vi "Control Panel No Objects.vi"(8 "error in (no error)":errorcluster) -> (0 "error out":errorcluster)   [LabVIEW 2009]
doc: "(Dynamic) A user-level application that simulates the physical front panel of the Instrument. Provide the user with buttons to manually control features of the instrument, and provide indicators of its current state."
uses:
  Areas.ctl
  Utility Classes/Readable/Channel Names.ctl
  Utility Classes/Readable/Channel Units.ctl
  Global/GPIB Numbers.vi
  <vilib>/Utility/error.llb/DialogType.ctl
  Spectrometer/JY-SPEX-TRIAX/controls.llb/Slits.ctl
  Synapse CCD.lvclass
  File IO/File IO.lvclass
  Spectrometer/JY-SPEX-TRIAX/JY-SPEX-TRIAX.lvlib
  Utility Classes/Readable/Readable.lvclass
panel:
  out "Resolution\n(nm/pixel)":dbl[unit] format="%#_3g"
  in  "File Name":path
  in  "Comments":string
  in  "Export\nPlot":bool
  in  "Cosmic Ray\nRemoval?":bool
  out "UnProcessed Spectra":T1(graph)
  in  "# to Average":u32
  in  "Averaging?":bool
  in  "Time Between Acq. (ms)":u32
  out "Spectrum":cluster{"Ramp Pattern":dbl[], "X array":dbl[]}[](graph)
  out "CCD State":string
  in  "Take Spectra":bool
  in  "Set CCD":bool
  in  "Set Grating":bool
  in  "stop":bool
  in  "Exit Slit":dbl[unit]
  in  "Entrance Slit":dbl[unit]
  out "Min":dbl[unit]
  out "Max":dbl[unit]
  in  "Center Wavelength":dbl[unit]
  in  "Grating":u16(ring) items=["1200 lines/mm - 500 nm Blaze", "1200 lines/mm - 750 nm Blaze", "600 lines/mm - 1000 nm Blaze"]
  in  "GAIN":u16(ring) caption="Device Name" items=["High Light", "Best Dynamic", "High Sensitivity"]
  in  "ADC":u16(ring) caption="Device Name" items=["   20 kHz", "1 MHz", "1 MHz Ultra"]
  in  "Integration time":dbl[unit]=0.01
  in  "Dark Subtract?":bool
  in  "Copy Actual to Set":bool
  in  "Populate Fields with Member Data":bool
  # "Must Set CCD after any change in this box"
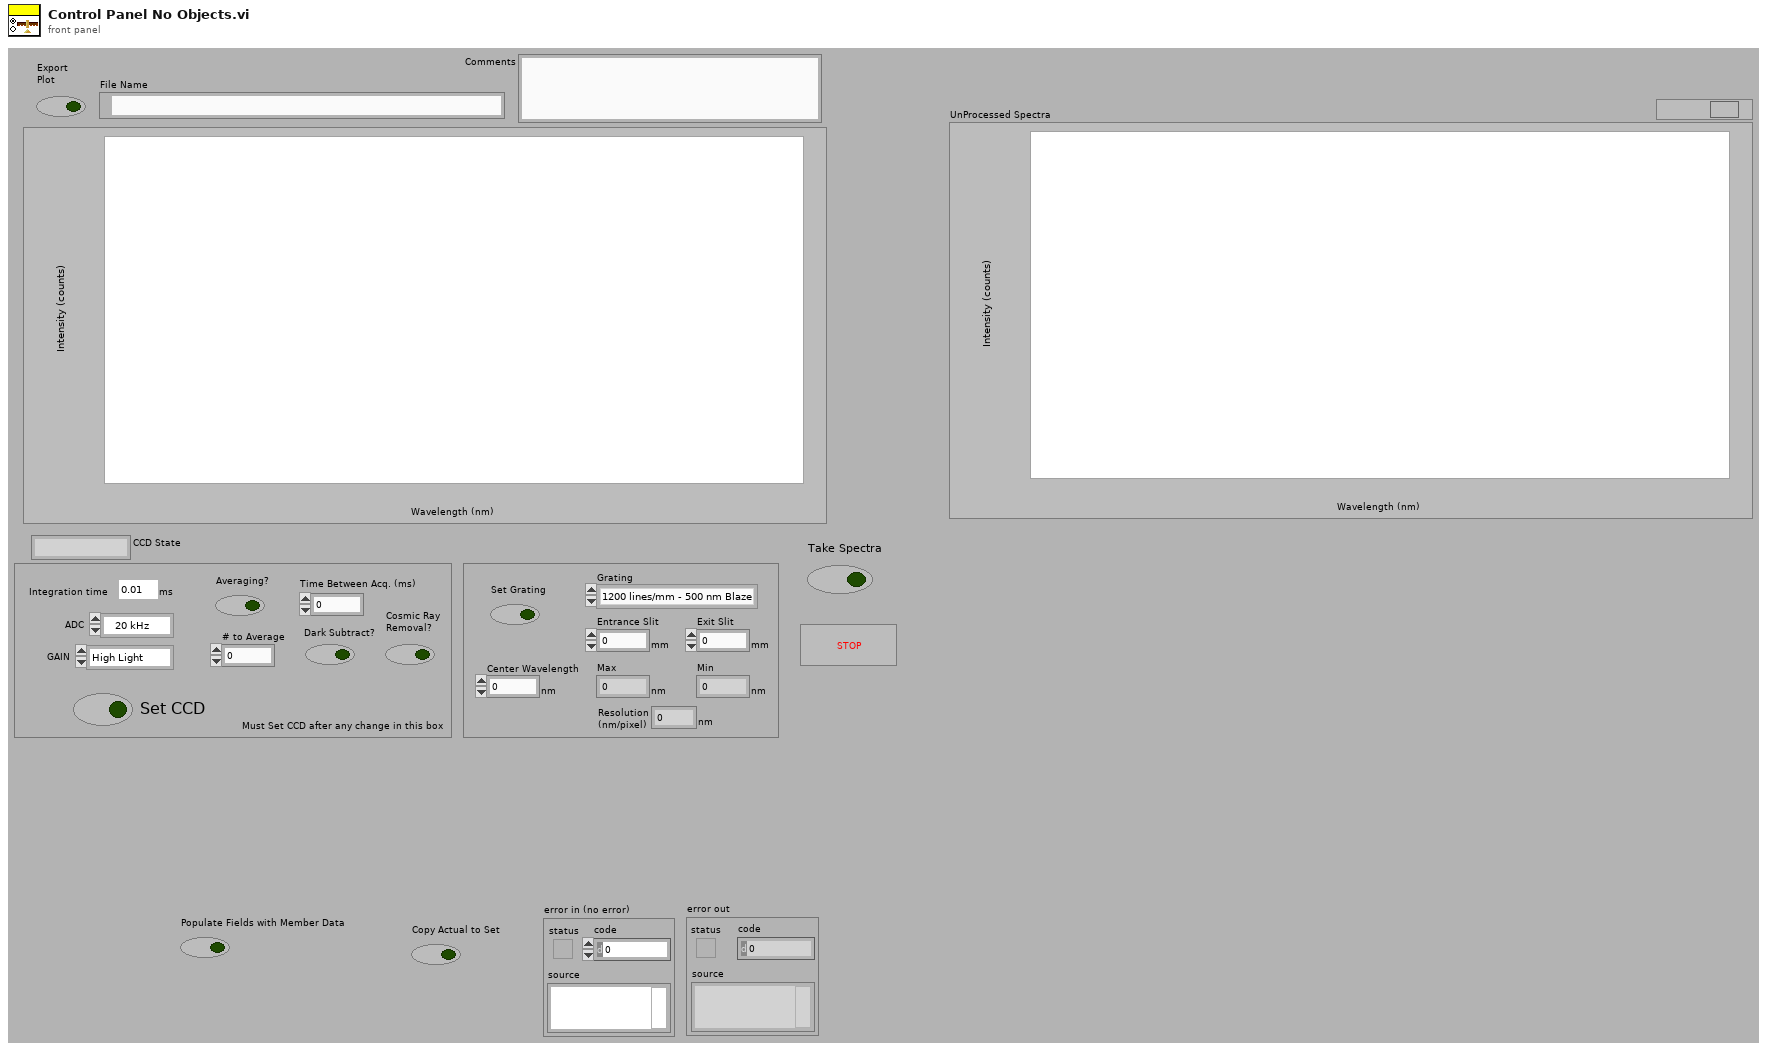
[diagram p1: front panel]
types:
  T1 = cluster{"Array of Wavelengths":dbl[], "Raw Data":i32[]}[]
  T2 = typedef "Synapse CCD.lvclass/Areas.ctl" = i32[][]
  T3 = typedef "Readable.lvclass/Channel Names.ctl" = string[]
  T4 = typedef "Readable.lvclass/Channel Units.ctl" = string[]
  T5 = cluster{"JYCCDLib.IJYCCDReqd":refnum<k7>, "JYMONOLib.IJYMonoReqd":refnum<k7>, "Integration time":dbl[unit], "ADC":u16, "GAIN":u16, "Areas":T2, "Most Recent Data Object":refnum<k7>, "Mono Properties":cluster{"Grating":u16, "Center Wavelength":dbl[unit], "Entrance Slit":dbl[unit], "Exit Slit":dbl[unit]}, "Coverage":cluster{"Max":dbl[unit], "Min":dbl[unit]}, "Multi-Acquisitions":cluster{"Dark Subtract?":bool, "Averaging?":bool, "Cosmic Ray Removal?":bool, "# to Average":u32, "Time Between Acq.":u32, "Acquisitions Control Array":bool[], "Raw Data":i32[][], "Processed Data":dbl[], "Array of Wavelengths":dbl[]}, "Channel Names":T3, "Channel Units":T4}
  T6 = typedef "DialogType.ctl" = u16
  T7 = typedef "GPIB Type Def.ctl" = cluster{"Name":string, "bus":dbl, "GPIB":dbl, "GPIB as string":string, "byte":i32, "VISA Resource Name":refnum<visa-resource-name>}
  T8 = typedef "JY-SPEX-TRIAX.lvlib/Slits.ctl" = enum16{"0 (Front/Axial Entrance)", "1 (Side/Lateral Entrance)", "2 (Front/Axial Exit)", "3 (Side/Lateral Exit)"}
  T9 = cluster{"Array of Wavelengths":dbl[], "Raw Data":i32[]}
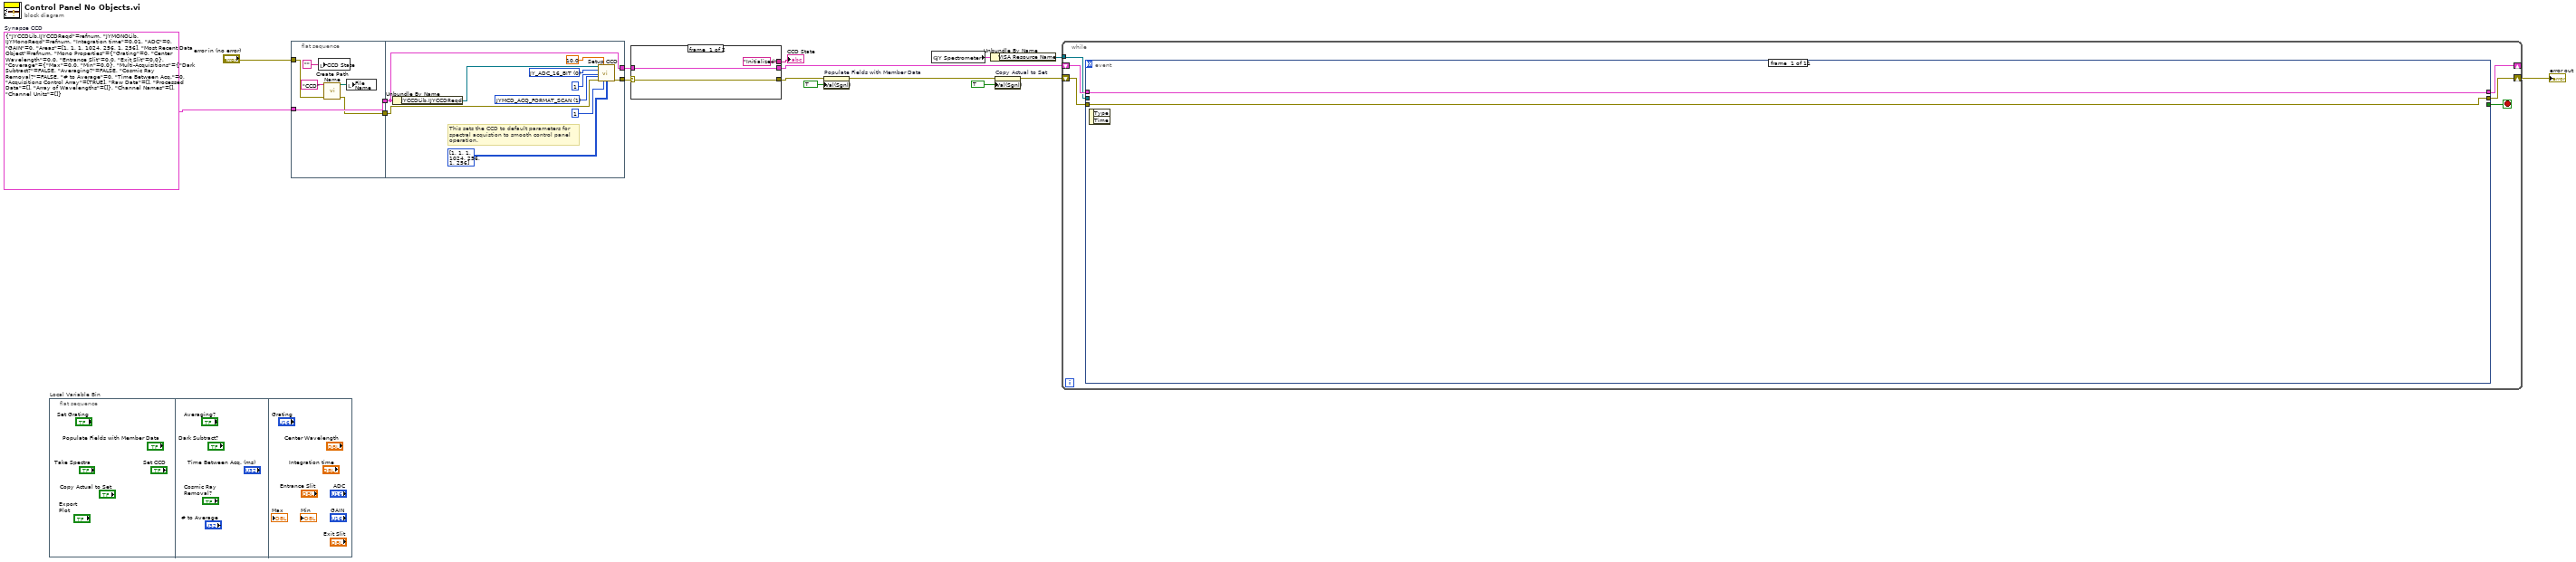
[diagram p0: block diagram]
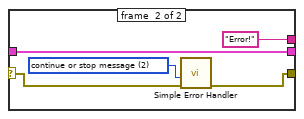
[diagram p2: hidden frame]
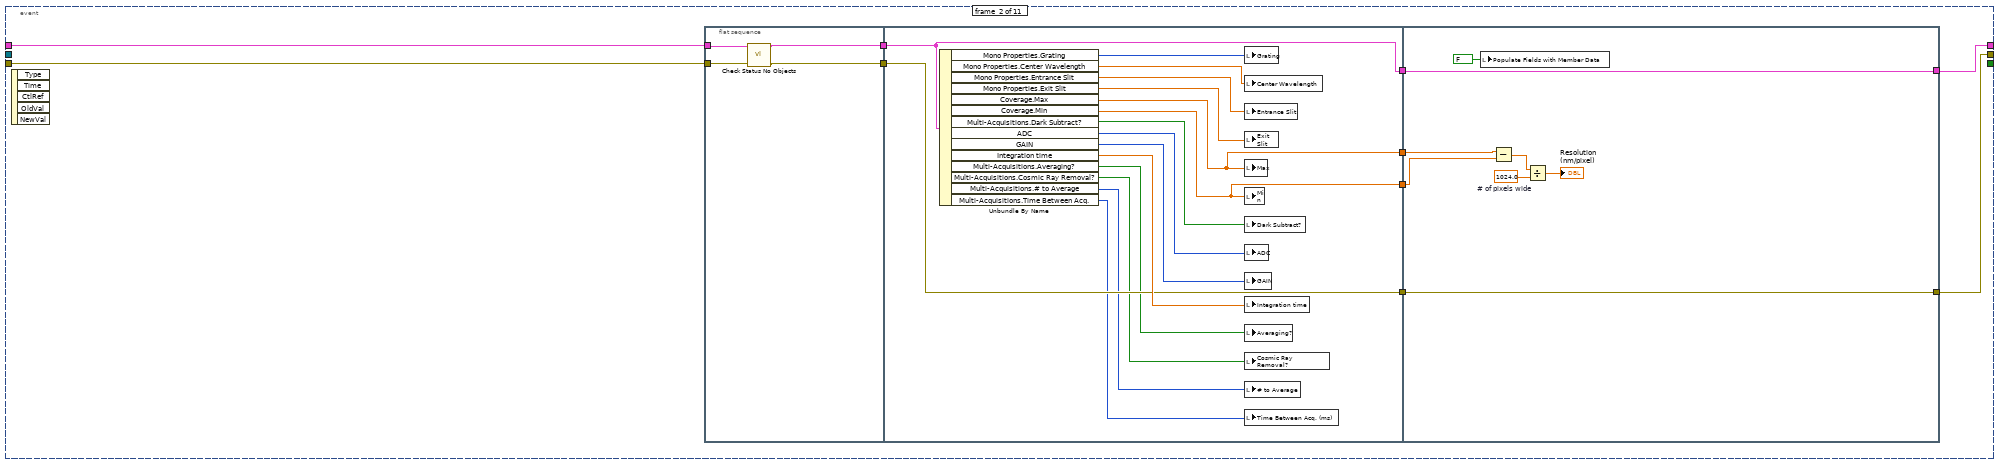
[diagram p3: hidden frame]
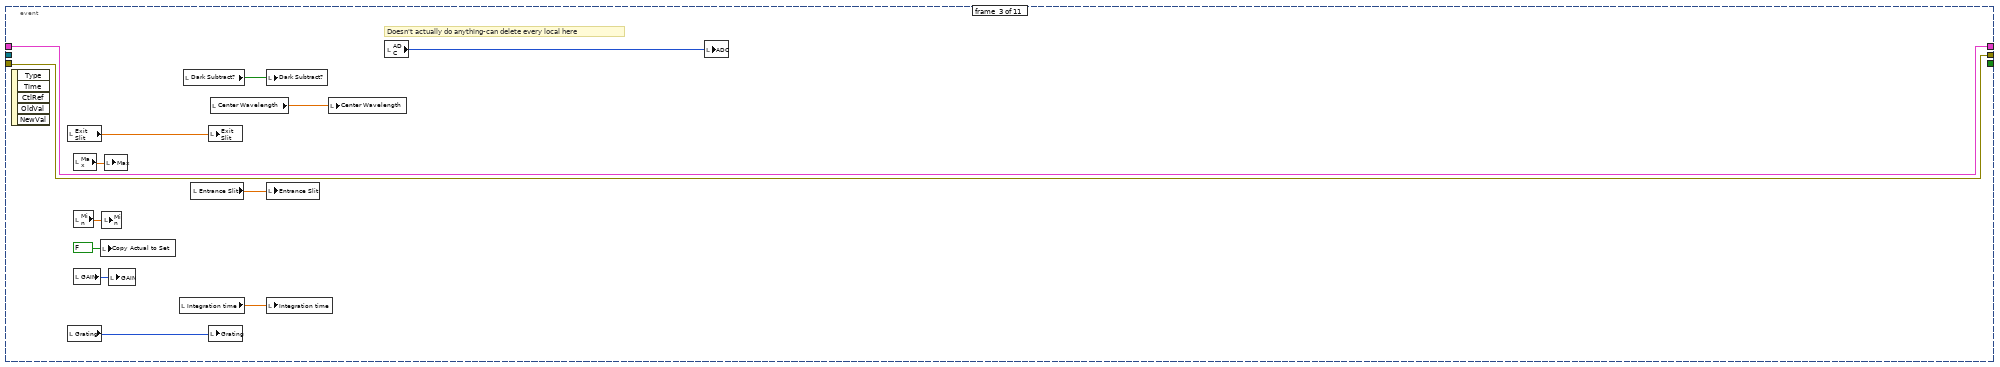
[diagram p4: hidden frame]
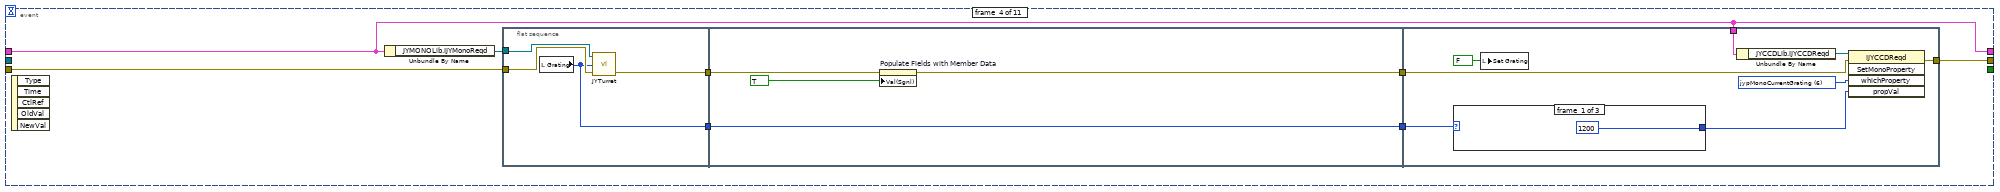
[diagram p5: hidden frame]
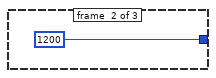
[diagram p6: hidden frame]
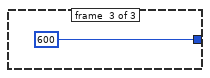
[diagram p7: hidden frame]
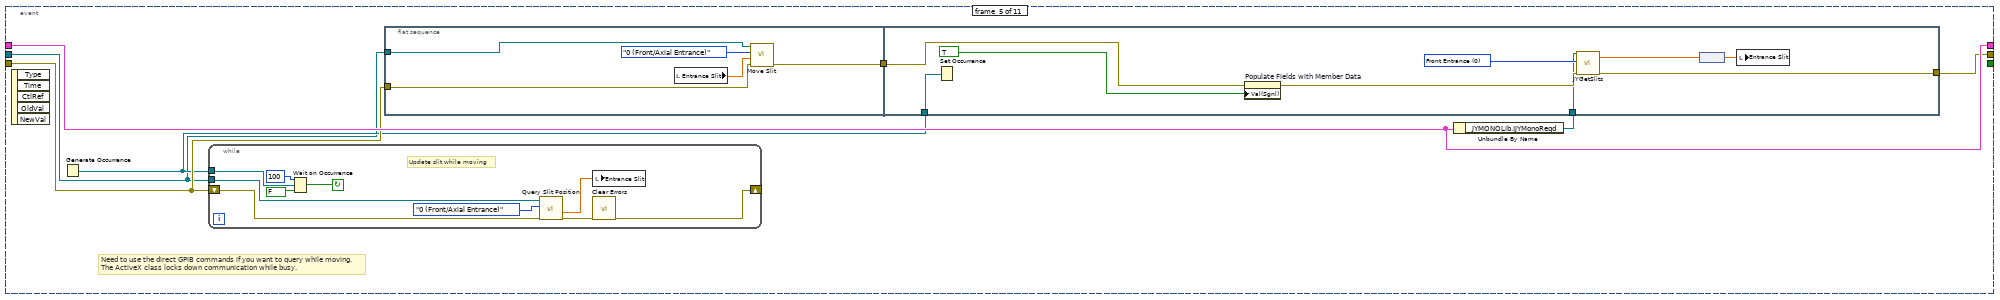
[diagram p8: hidden frame]
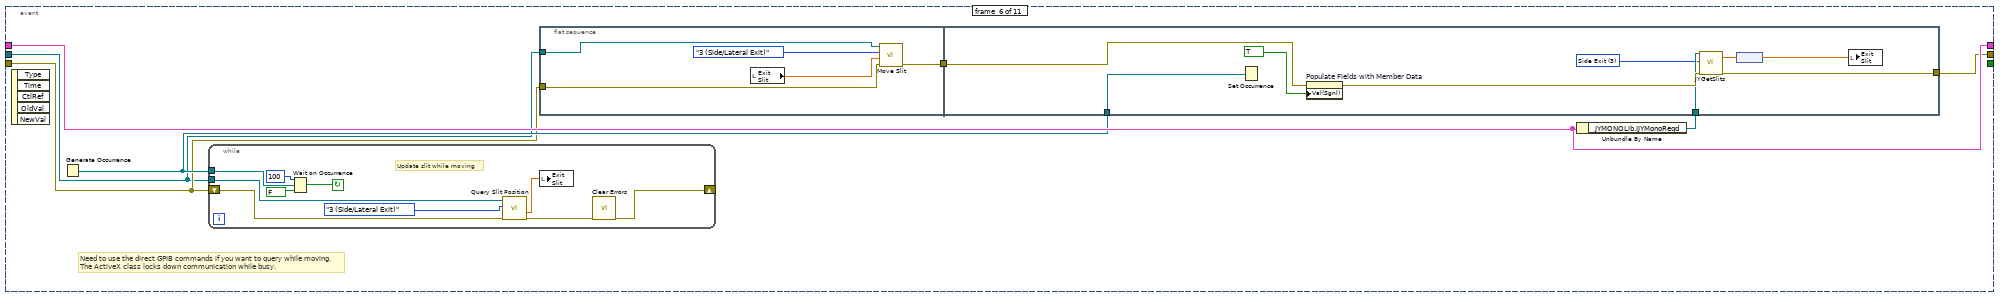
[diagram p9: hidden frame]
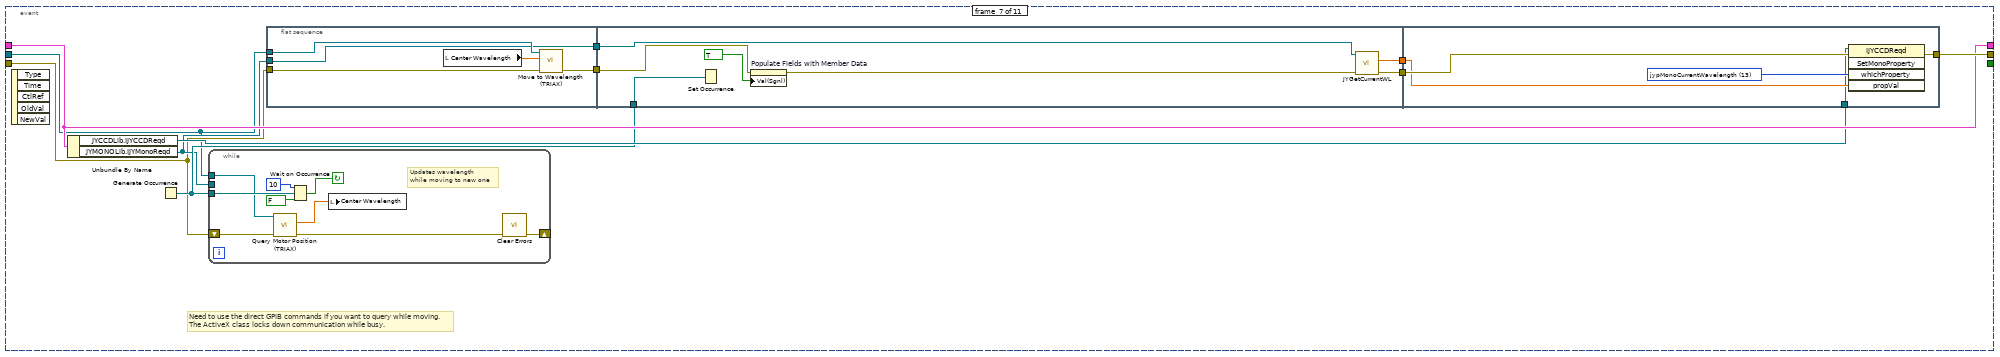
[diagram p10: hidden frame]
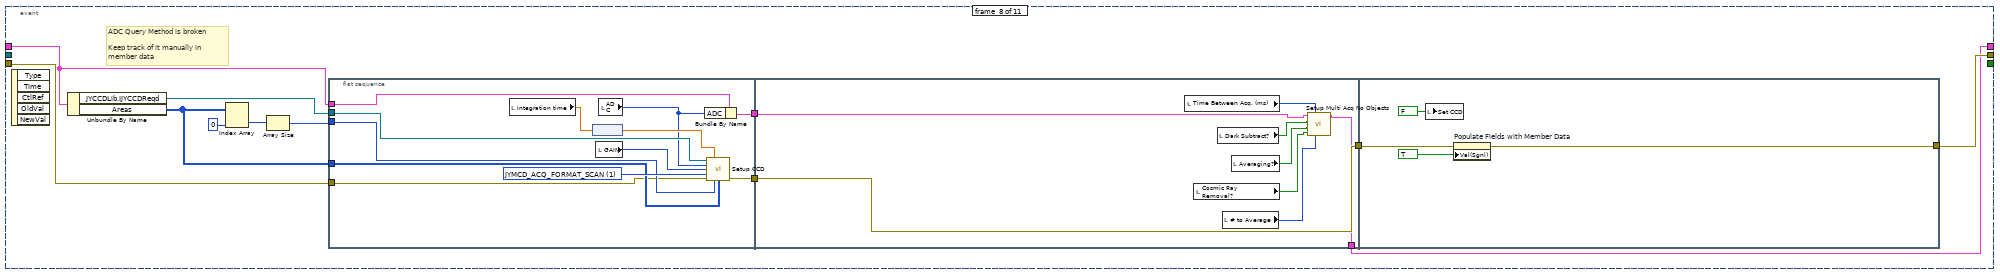
[diagram p11: hidden frame]
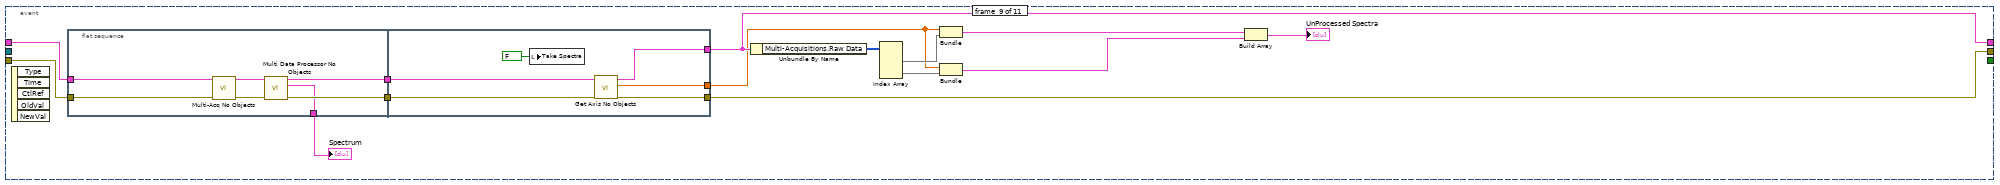
[diagram p12: hidden frame]
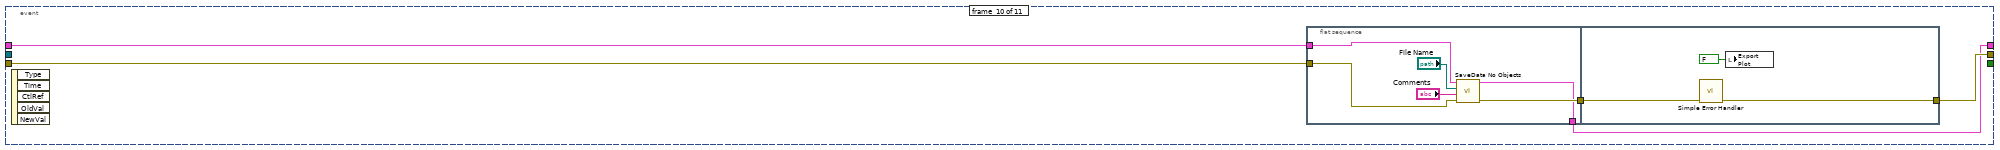
[diagram p13: hidden frame]
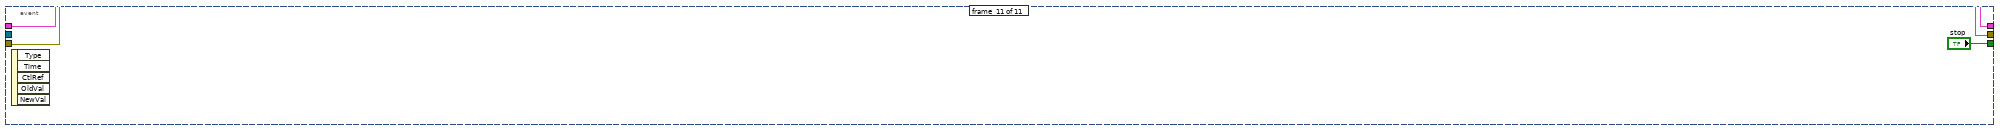
[diagram p14: hidden frame]
diagram:
  w3 = T5 {"JYCCDLib.IJYCCDReqd"=refnum, "JYMONOLib.IJYMonoReqd"=refnum, "Integration time"=0.01, "ADC"=0, "GAIN"=0, "Areas"=[[1, 1, 1, 1024, 256, 1, 256]], "Most Recent Data Object"=refnum, "Mono Properties"={"Grating"=0, "Center Wavelength"=0.0, "Entrance Slit"=0.0, "Exit Slit"=0.0}, "Coverage"={"Max"=0.0, "Min"=0.0}, "Multi-Acquisitions"={"Dark Subtract?"=FALSE, "Averaging?"=FALSE, "Cosmic Ray Removal?"=FALSE, "# to Average"=0, "Time Between Acq."=0, "Acquisitions Control Array"=[TRUE], "Raw Data"=[], "Processed Data"=[], "Array of Wavelengths"=[]}, "Channel Names"=[], "Channel Units"=[]}  # Synapse CCD
  n1 = flat-sequence "Local Variable Bin" {
    frame #0 {
    }
    frame #1 {
    }
    frame #2 {
    }
  }
  n2 = flat-sequence {
    tunnel: "error in (no error)" -> [w22]
    tunnel: [w18] -> w7
    tunnel: w3 -> [w18]
    tunnel: [w17] -> w2
    tunnel: [w32] -> w11
    tunnel: [w23] -> w12
    tunnel: w7 -> [w32]
    tunnel: w2 -> [w26]
    frame #0 {
      n3 = local write "CCD State"("") -> ()
      n4 = call "Create Path Name.vi"("error in"=w22, "filename"="CCD") -> ("error out"=w17:errorcluster, "path"=w20:path)  [unwired: 4 out]
      n5 = local write "File Name"(w20) -> ()
    }
    frame #1 {
      w27 = 1 items=["JYMCD_ACQ_FORMAT_IMAGE", "JYMCD_ACQ_FORMAT_SCAN"] ("Acquisition type")
      w29 = 0 items=["JY_ADC_16_BIT", "JY_ADC_14_BIT", "JY_ADC_18_BIT"] ("Select ADC")
      # "This sets the CCD to default parameters for\nspectral acquistion to smooth control panel\noperation."
      n6 = Unbundle By Name(w32) -> ("JYCCDLib.IJYCCDReqd"=w31:refnum<k7>)
      n7 = call "Setup CCD.vi"("IJYCCDReqd In"=w31, "Integration time(ms)"=10.0 ("IntegrationTime"), "Select ADC"=w29, "Gain"=1, "Acquisition type"=w27, "error in (no error)"=w26, "numAreas"=1, "areas :"=T2 [[1, 1, 1, 1024, 256, 1, 256]] ("Areas")) -> ("error out"=w23:errorcluster)  [unwired: 5 in, 2 out]
    }
  }
  n8 = case shown="No Error" w12 {
    selector: w12 -> [w34 w38]
    tunnel: w11 -> [w35 w40]
    tunnel: [w35 w40] -> w10
    tunnel: [w34 w37] -> w9
    tunnel: ["Initialized" ("String") "Error!" ("String")] -> w8
    frame #0 {
    }
    frame #1 {
      w36 = T6 2 items=["no dialog", "OK message", "continue or stop message", "OK message + warnings", "continue/stop + warnings"] ("type of dialog (OK msg:1)")
      n9 = call <vilib>:"Simple Error Handler.vi"("type of dialog (OK msg:1)"=w36, "error in (no error)"=w38) -> ("error out"=w37:errorcluster)  [unwired: 3 in, 4 out]
    }
  }
  "CCD State" <- w8
  n10 = property on="Populate Fields with Member Data" class="Bool (strict)"(error in=w9, "Val(Sgnl)"=TRUE ("Value (Signaling)")) -> (error out=w16:errorcluster)  [unwired: 1 in, 1 out]
  n11 = global read "GPIB Numbers.vi" "JY Spectrometer"() -> (w6:T7)
  n12 = Unbundle By Name(w6) -> ("VISA Resource Name"=w5:refnum<visa-resource-name>)
  n13 = property on="Copy Actual to Set" class="Bool (strict)"(error in=w16, "Val(Sgnl)"=TRUE ("Value (Signaling)")) -> (error out=w15:errorcluster)  [unwired: 1 in, 1 out]
  n14 = while {
    shift-right: [w44] -> w1
    shift-left: w15 -> [w45]
    shift-right: [w43] -> _
    shift-left: w10 -> [w46]
    tunnel: w5 -> [w41]
    stop <- w42 stop-if-true
    n15 = event shown="[9] \"Export\nPlot\": Value Change" {
      selector: _ -> [_ _ _ _ _ _ _ _ _ _ _]
      dyn-events: _ -> [_ _ _ _ _ _ _ _ _ _ _]
      timeout: _ -> [_ _ _ _ _ _ _ _ _ _ _]
      tunnel: w46 -> [w48 w58 w88 w100 w132 w163 w195 w227 w271 w292 w304]
      tunnel: w45 -> [w47 w56 w89 w106 w130 w160 w190 w233 w275 w293 w303]
      tunnel: [w47 w55 w89 w105 w131 w162 w199 w232 w272 w291 w303] -> w44
      tunnel: [w48 w57 w88 w100 w132 w163 w195 w228 w270 w290 w304] -> w43
      tunnel: [_ _ _ _ _ _ _ _ _ _ "stop"] -> w42
      tunnel: w41 -> [_ _ _ _ w128 w158 w189 _ _ _ _]
      event #0 {
        n16 = event-data() -> ()  [unwired: 1 in, 2 out]
      }
      event #1 {
        n17 = event-data() -> ()  [unwired: 1 in, 5 out]
        n18 = flat-sequence {
          tunnel: w56 -> [w59]
          tunnel: w58 -> [w62]
          tunnel: [w61] -> w52
          tunnel: [w60] -> w51
          tunnel: [w70] -> w54
          tunnel: [w69] -> w53
          tunnel: w52 -> [w70]
          tunnel: w51 -> [w69]
          tunnel: [w64] -> w50
          tunnel: [w63] -> w49
          tunnel: [w85] -> w55
          tunnel: [w86] -> w57
          tunnel: w54 -> [w86]
          tunnel: w53 -> [w85]
          tunnel: w50 -> [w83]
          tunnel: w49 -> [w82]
          frame #0 {
            n19 = call "Check Status No Objects.vi"("error in (no error)"=w59, "Synapse CCD in"=w62) -> ("error out"=w60:errorcluster, "Synapse CCD out"=w61:T5)  [unwired: 6 in, 2 out]
          }
          frame #1 {
            n20 = Unbundle By Name(w70) -> ("Mono Properties.Grating"=w78:u16, "Mono Properties.Center Wavelength"=w77:dbl[unit], "Mono Properties.Entrance Slit"=w76:dbl[unit], "Mono Properties.Exit Slit"=w75:dbl[unit], "Coverage.Max"=w64:dbl[unit], "Coverage.Min"=w63:dbl[unit], "Multi-Acquisitions.Dark Subtract?"=w74:bool, "ADC"=w73:u16, "GAIN"=w72:u16, "Integration time"=w71:dbl[unit], "Multi-Acquisitions.Averaging?"=w65:bool, "Multi-Acquisitions.Cosmic Ray Removal?"=w66:bool, "Multi-Acquisitions.# to Average"=w67:u32, "Multi-Acquisitions.Time Between Acq."=w68:u32)
            n21 = local write "Grating"(w78) -> ()
            n22 = local write "Center Wavelength"(w77) -> ()
            n23 = local write "Entrance Slit"(w76) -> ()
            n24 = local write "Exit Slit"(w75) -> ()
            n25 = local write "Max"(w64) -> ()
            n26 = local write "Min"(w63) -> ()
            n27 = local write "Dark Subtract?"(w74) -> ()
            n28 = local write "ADC"(w73) -> ()
            n29 = local write "GAIN"(w72) -> ()
            n30 = local write "Integration time"(w71) -> ()
            n31 = local write "Averaging?"(w65) -> ()
            n32 = local write "Cosmic Ray\nRemoval?"(w66) -> ()
            n33 = local write "# to Average"(w67) -> ()
            n34 = local write "Time Between Acq. (ms)"(w68) -> ()
          }
          frame #2 {
            w80 = 1024.0  # # of pixels wide
            n35 = local write "Populate Fields with Member Data"(FALSE ("Populate Fields with Member Data")) -> ()
            n36 = Subtract(x=w83, y=w82) -> (x-y=w81:dbl[unit])
            n37 = Divide(x=w81, y=w80) -> (x/y=→"Resolution\n(nm/pixel)":dbl[unit])
          }
        }
      }
      event #2 {
        # "Doesn't actually do anything-can delete every local here"
        n38 = event-data() -> ()  [unwired: 1 in, 5 out]
        n39 = local read "Exit Slit"() -> (w94:dbl[unit])
        n40 = local read "Grating"() -> (w92:u16)
        n41 = local read "Max"() -> (w90:dbl[unit])
        n42 = local read "Min"() -> (w96:dbl[unit])
        n43 = local read "GAIN"() -> (w93:u16)
        n44 = local write "Copy Actual to Set"(FALSE ("Copy Actual to Set")) -> ()
        n45 = local write "Min"(w96) -> ()
        n46 = local write "Max"(w90) -> ()
        n47 = local write "GAIN"(w93) -> ()
        n48 = local read "Integration time"() -> (w91:dbl[unit])
        n49 = local read "Dark Subtract?"() -> (w97:bool)
        n50 = local read "Entrance Slit"() -> (w95:dbl[unit])
        n51 = local write "Exit Slit"(w94) -> ()
        n52 = local write "Grating"(w92) -> ()
        n53 = local read "Center Wavelength"() -> (w98:dbl[unit])
        n54 = local write "Dark Subtract?"(w97) -> ()
        n55 = local write "Entrance Slit"(w95) -> ()
        n56 = local write "Integration time"(w91) -> ()
        n57 = local write "Center Wavelength"(w98) -> ()
        n58 = local read "ADC"() -> (w99:u16)
        n59 = local write "ADC"(w99) -> ()
      }
      event #3 {
        n60 = event-data() -> ()  [unwired: 1 in, 5 out]
        n61 = Unbundle By Name(w100) -> ("JYMONOLib.IJYMonoReqd"=w107:refnum<k7>)
        n62 = flat-sequence {
          tunnel: w107 -> [w111]
          tunnel: w106 -> [w110]
          tunnel: [w109] -> w104
          tunnel: [w108] -> w102
          tunnel: w104 -> [w114]
          tunnel: [w113] -> w103
          tunnel: w102 -> [w113]
          tunnel: [w112] -> w101
          tunnel: [w122] -> w105
          tunnel: w103 -> [w117]
          tunnel: w101 -> [w120]
          tunnel: w100 -> [w119]
          frame #0 {
            n63 = local read "Grating"() -> (w108:u16)
            n64 = call "JYTurret.vi"("error in (no error)"=w110, "Grating Index"=w108, "JYMONOLib.IJYMonoReqd In"=w111) -> ("error out"=w109:errorcluster)  [unwired: 2 out]
          }
          frame #1 {
            n65 = property on="Populate Fields with Member Data" class="Bool (strict)"(error in=w114, "Val(Sgnl)"=TRUE ("Value (Signaling)")) -> (error out=w112:errorcluster)  [unwired: 1 in, 1 out]
          }
          frame #2 {
            w121 = 6 items=["jyUndefined", "jypMonoLinearDispersion", "jypMonoBacklashAmount", "jypMonoStepsPerUnit", "jypMonoBaseUnits", "jypMonoBaseGrating", "jypMonoCurrentGrating", "jypMonoMaxLimit", "jypMonoMinLimit", "jypMonoTiltAngle", "jypMonoIncludedAngle", "jypMonoFocalLength", "jypMonoOrder", "jypMonoCurrentWavelength", "jypMonoMCDWavelengthDirection", "jypBandpassUnits", "jypSlitMaxLimit", "jypSlitMinLimit", "jypSlitBackLashAmount", "jypSlitBaseUnits", "jypSlitStepsPerUnit", "jypLaserLine", "jypTotalHardwarePropertiesPlusOne", "jypCurrentTurretPosition"] ("whichProperty")
            n66 = case shown="2" w117 {
              tunnel: [u16 1200 u16 1200 u16 600] -> w116
              frame #0 {
              }
              frame #1 {
              }
              frame #2 {
              }
            }
            n67 = local write "Set Grating"(FALSE ("Set Spectrometer")) -> ()
            n68 = Unbundle By Name(w119) -> ("JYCCDLib.IJYCCDReqd"=w123:refnum<k7>)
            n69 = invoke class="IJYCCDReqd" method="SetMonoProperty"(reference=w123, error in=w120, "whichProperty"=w121, "propVal"=w116) -> (error out=w122:errorcluster)  [unwired: 1 in, 4 out]
          }
        }
      }
      event #4 {
        # "Need to use the direct GPIB commands if you want to query while moving.\nThe ActiveX class locks down communication while busy."
        n70 = event-data() -> ()  [unwired: 1 in, 5 out]
        n71 = Generate Occurrence() -> (w129:refnum<k4>)
        n72 = while {
          tunnel: w129 -> [w143]
          shift-right: [w134] -> _
          shift-left: w130 -> [w139]
          tunnel: w128 -> [w138]
          stop <- w142 continue-if-true
          # "Update slit while moving"
          n73 = Wait on Occurrence(1:FALSE ("ignore previous (T)"), 2:w143, 3:100 ("ms timeout (-1)")) -> (0:w142:bool)
          n74 = call "Query Slit Position.vi"("error in (no error)"=w139, "Slit (Front/Axial Entrance)"=Slits."0 (Front/Axial Entrance)", "VISA resource name"=w138) -> ("error out"=w135:errorcluster, "Slit Position"=w136:dbl[unit])  [unwired: 6 in, 1 out]
          n75 = local write "Entrance Slit"(w136) -> ()
          n76 = call <vilib>:"Clear Errors.vi"("error in (no error)"=w135) -> ("error out"=w134:errorcluster)  [unwired: 6 in]
        }
        n77 = flat-sequence {
          tunnel: w130 -> [w147]
          tunnel: [w146] -> w133
          tunnel: w128 -> [w144]
          tunnel: w133 -> [w156]
          tunnel: [w153] -> w131
          tunnel: w129 -> [w155]
          tunnel: w127 -> [w151]
          frame #0 {
            n78 = local read "Entrance Slit"() -> (w148:dbl[unit])
            n79 = call "Move Slit.vi"("error in (no error)"=w147, "Desired Slit Position"=w148, "Slit (Front/Axial Entrance)"=Slits."0 (Front/Axial Entrance)", "VISA resource name"=w144) -> ("error out"=w146:errorcluster)  [unwired: 6 in, 1 out]
          }
          frame #1 {
            w152 = u16 0 items=["Front Entrance", "Side Entrance", "Front Exit", "Side Exit", "First Intermediate", "Second Intermediate"] ("Slit")
            n80 = Set Occurrence(w155) -> ()
            n81 = property on="Populate Fields with Member Data" class="Bool (strict)"(error in=w156, "Val(Sgnl)"=TRUE ("Value (Signaling)")) -> (error out=w154:errorcluster)  [unwired: 1 in, 1 out]
            n82 = call "JYGetSlits.vi"("MonoRefNum IN"=w151, "Slit"=w152, "error in (no error)"=w154) -> ("Slit Width"=w149:dbl, "error out"=w153:errorcluster)  [unwired: 13 in, 2 out]
            n83 = node(w149) -> (w150:dbl[unit])
            n84 = local write "Entrance Slit"(w150) -> ()
          }
        }
        n85 = Unbundle By Name(w132) -> ("JYMONOLib.IJYMonoReqd"=w127:refnum<k7>)
      }
      event #5 {
        # "Need to use the direct GPIB commands if you want to query while moving.\nThe ActiveX class locks down communication while busy."
        n86 = event-data() -> ()  [unwired: 1 in, 5 out]
        n87 = Generate Occurrence() -> (w161:refnum<k4>)
        n88 = while {
          tunnel: w161 -> [w174]
          shift-right: [w165] -> _
          shift-left: w160 -> [w169]
          tunnel: w158 -> [w168]
          stop <- w172 continue-if-true
          # "Update slit while moving"
          n89 = Wait on Occurrence(1:FALSE ("ignore previous (T)"), 2:w174, 3:100 ("ms timeout (-1)")) -> (0:w172:bool)
          n90 = call "Query Slit Position.vi"("error in (no error)"=w169, "Slit (Front/Axial Entrance)"=Slits."3 (Side/Lateral Exit)", "VISA resource name"=w168) -> ("error out"=w166:errorcluster, "Slit Position"=w170:dbl[unit])  [unwired: 6 in, 1 out]
          n91 = local write "Exit Slit"(w170) -> ()
          n92 = call <vilib>:"Clear Errors.vi"("error in (no error)"=w166) -> ("error out"=w165:errorcluster)  [unwired: 6 in]
        }
        n93 = flat-sequence {
          tunnel: w160 -> [w178]
          tunnel: [w177] -> w164
          tunnel: w158 -> [w176]
          tunnel: w164 -> [w187]
          tunnel: [w184] -> w162
          tunnel: w161 -> [w186]
          tunnel: w159 -> [w183]
          frame #0 {
            n94 = local read "Exit Slit"() -> (w179:dbl[unit])
            n95 = call "Move Slit.vi"("error in (no error)"=w178, "Desired Slit Position"=w179, "Slit (Front/Axial Entrance)"=Slits."3 (Side/Lateral Exit)", "VISA resource name"=w176) -> ("error out"=w177:errorcluster)  [unwired: 6 in, 1 out]
          }
          frame #1 {
            w182 = u16 3 items=["Front Entrance", "Side Entrance", "Front Exit", "Side Exit", "First Intermediate", "Second Intermediate"] ("Slit")
            n96 = Set Occurrence(w186) -> ()
            n97 = property on="Populate Fields with Member Data" class="Bool (strict)"(error in=w187, "Val(Sgnl)"=TRUE ("Value (Signaling)")) -> (error out=w185:errorcluster)  [unwired: 1 in, 1 out]
            n98 = call "JYGetSlits.vi"("MonoRefNum IN"=w183, "Slit"=w182, "error in (no error)"=w185) -> ("Slit Width"=w181:dbl, "error out"=w184:errorcluster)  [unwired: 13 in, 2 out]
            n99 = node(w181) -> (w180:dbl[unit])
            n100 = local write "Exit Slit"(w180) -> ()
          }
        }
        n101 = Unbundle By Name(w163) -> ("JYMONOLib.IJYMonoReqd"=w159:refnum<k7>)
      }
      event #6 {
        # "Need to use the direct GPIB commands if you want to query while moving.\nThe ActiveX class locks down communication while busy."
        n102 = event-data() -> ()  [unwired: 1 in, 5 out]
        n103 = Unbundle By Name(w195) -> ("JYCCDLib.IJYCCDReqd"=w193:refnum<k7>, "JYMONOLib.IJYMonoReqd"=w191:refnum<k7>)
        n104 = Generate Occurrence() -> (w192:refnum<k4>)
        n105 = while {
          tunnel: w192 -> [w208]
          tunnel: w191 -> [_]
          shift-right: [w204] -> _
          shift-left: w190 -> [w203]
          tunnel: w189 -> [w200]
          stop <- w206 continue-if-true
          # "Updates wavelength\nwhile moving to new one"
          n106 = call "Query Motor Position (TRIAX).vi"("error in (no error)"=w203, "VISA resource name"=w200) -> ("error out"=w202:errorcluster, "wavelength"=w201:dbl[unit])  [unwired: 7 in, 1 out]
          n107 = Wait on Occurrence(1:FALSE ("ignore previous (T)"), 2:w208, 3:10 ("ms timeout (-1)")) -> (0:w206:bool)
          n108 = local write "Center Wavelength"(w201) -> ()
          n109 = call <vilib>:"Clear Errors.vi"("error in (no error)"=w202) -> ("error out"=w204:errorcluster)  [unwired: 6 in]
        }
        n110 = flat-sequence {
          tunnel: w191 -> [w209]
          tunnel: w190 -> [w212]
          tunnel: [w211] -> w198
          tunnel: [w209] -> w194
          tunnel: w189 -> [w210]
          tunnel: w198 -> [w219]
          tunnel: [w217] -> w197
          tunnel: [w215] -> w196
          tunnel: w194 -> [w216]
          tunnel: w192 -> [w214]
          tunnel: [w222] -> w199
          tunnel: w197 -> [w225]
          tunnel: w196 -> [w223]
          tunnel: w193 -> [w221]
          frame #0 {
            n111 = local read "Center Wavelength"() -> (w213:dbl[unit])
            n112 = call "Move to Wavelength (TRIAX).vi"("error in (no error)"=w212, "Target wavelength"=w213, "VISA resource name"=w210) -> ("error out"=w211:errorcluster)  [unwired: 7 in, 1 out]
          }
          frame #1 {
            n113 = Set Occurrence(w214) -> ()
            n114 = property on="Populate Fields with Member Data" class="Bool (strict)"(error in=w219, "Val(Sgnl)"=TRUE ("Value (Signaling)")) -> (error out=w218:errorcluster)  [unwired: 1 in, 1 out]
            n115 = call "JYGetCurrentWL.vi"("error in (no error)"=w218, "JYMONOLib.IJYMonoReqd In"=w216) -> ("error out"=w217:errorcluster, "Current WL"=w215:dbl)  [unwired: 6 in, 2 out]
          }
          frame #2 {
            w224 = 13 items=["jyUndefined", "jypMonoLinearDispersion", "jypMonoBacklashAmount", "jypMonoStepsPerUnit", "jypMonoBaseUnits", "jypMonoBaseGrating", "jypMonoCurrentGrating", "jypMonoMaxLimit", "jypMonoMinLimit", "jypMonoTiltAngle", "jypMonoIncludedAngle", "jypMonoFocalLength", "jypMonoOrder", "jypMonoCurrentWavelength", "jypMonoMCDWavelengthDirection", "jypBandpassUnits", "jypSlitMaxLimit", "jypSlitMinLimit", "jypSlitBackLashAmount", "jypSlitBaseUnits", "jypSlitStepsPerUnit", "jypLaserLine", "jypTotalHardwarePropertiesPlusOne", "jypCurrentTurretPosition"] ("whichProperty")
            n116 = invoke class="IJYCCDReqd" method="SetMonoProperty"(reference=w221, error in=w225, "whichProperty"=w224, "propVal"=w223) -> (error out=w222:errorcluster)  [unwired: 1 in, 4 out]
          }
        }
      }
      event #7 {
        # "ADC Query Method is broken\n\nKeep track of it manually in \nmember data"
        n117 = event-data() -> ()  [unwired: 1 in, 5 out]
        n118 = Unbundle By Name(w227) -> ("JYCCDLib.IJYCCDReqd"=w234:refnum<k7>, "Areas"=w235:T2)
        n119 = Index Array(array=w235, index (col)=0 ("index (row)")) -> (element=w236:i32[])  [unwired: 1 in]
        n120 = Array Size(array=w236) -> (size(s)=w237:i32)
        n121 = flat-sequence {
          tunnel: w237 -> [w248]
          tunnel: w235 -> [w247]
          tunnel: w234 -> [w244]
          tunnel: w233 -> [w243]
          tunnel: [w242] -> w231
          tunnel: w227 -> [w240]
          tunnel: [w239] -> w226
          tunnel: w231 -> [w257]
          tunnel: [w257] -> w229
          tunnel: [w256] -> w228
          tunnel: w226 -> [w250]
          tunnel: [w258] -> w232
          tunnel: w229 -> [w259]
          frame #0 {
            w249 = 1 items=["JYMCD_ACQ_FORMAT_IMAGE", "JYMCD_ACQ_FORMAT_SCAN"] ("Acquisition type")
            n122 = local read "Integration time"() -> (w246:dbl[unit])
            n123 = node(w246) -> (w241:dbl)
            n124 = local read "GAIN"() -> (w245:u16)
            n125 = local read "ADC"() -> (w238:u16)
            n126 = Bundle By Name(cluster=w240, "ADC"=w238) -> (w239:T5)
            n127 = call "Setup CCD.vi"("IJYCCDReqd In"=w244, "Integration time(ms)"=w241, "Select ADC"=w238, "Gain"=w245, "Acquisition type"=w249, "error in (no error)"=w243, "numAreas"=w248, "areas :"=w247) -> ("error out"=w242:errorcluster)  [unwired: 5 in, 2 out]
          }
          frame #1 {
            n128 = local read "Time Between Acq. (ms)"() -> (w255:u32)
            n129 = local read "Cosmic Ray\nRemoval?"() -> (w253:bool)
            n130 = local read "Dark Subtract?"() -> (w251:bool)
            n131 = local read "# to Average"() -> (w254:u32)
            n132 = local read "Averaging?"() -> (w252:bool)
            n133 = call "Setup Multi Acq No Objects.vi"("# of Scans"=w254, "Time Between Acq (ms)"=w255, "Cosmic Ray Removal?"=w253, "Averaging?"=w252, "Dark Subtract?"=w251, "Synapse CCD in"=w250) -> ("Synapse CCD out"=w256:T5)  [unwired: 5 in]
          }
          frame #2 {
            n134 = local write "Set CCD"(FALSE ("Set CCD")) -> ()
            n135 = property on="Populate Fields with Member Data" class="Bool (strict)"(error in=w259, "Val(Sgnl)"=TRUE) -> (error out=w258:errorcluster)  [unwired: 1 in, 1 out]
          }
        }
      }
      event #8 {
        n136 = event-data() -> ()  [unwired: 1 in, 5 out]
        n137 = flat-sequence {
          tunnel: w275 -> [w281]
          tunnel: w271 -> [w282]
          tunnel: [w276] -> w274
          tunnel: [w278] -> w273
          tunnel: [w277] -> w268
          tunnel: w274 -> [w285]
          tunnel: [w284] -> w270
          tunnel: w273 -> [w286]
          tunnel: [w287] -> w272
          tunnel: [w283] -> w264
          frame #0 {
            n138 = call "Multi-Acq No Objects.vi"("error in"=w281, "Synapse CCD in"=w282) -> ("error out"=w279:errorcluster, "Synapse CCD out"=w280:T5)  [unwired: 8 in]
            n139 = call "Multi Data Processor No Objects.vi"("error in (no error)"=w279, "Synapse CCD in"=w280) -> ("error out"=w278:errorcluster, "Processed Spectrum"=w277:cluster{"Ramp Pattern":dbl[], "X array":dbl[]}[], "Synapse CCD out"=w276:T5)  [unwired: 6 in, 1 out]
          }
          frame #1 {
            n140 = local write "Take Spectra"(FALSE ("Take Spectra")) -> ()
            n141 = call "Get Axis No Objects.vi"("error in (no error)"=w286, "Synapse CCD in"=w285) -> ("error out"=w287:errorcluster, "Array of Wavelengths"=w283:dbl[], "Synapse CCD out"=w284:T5)  [unwired: 7 in]
          }
        }
        n142 = Unbundle By Name(w270) -> ("Multi-Acquisitions.Raw Data"=w269:i32[][])
        n143 = Index Array(array=w269) -> (element #1=w267:i32[], element #2=w263:i32[])  [unwired: 4 in]
        n144 = Bundle("Array of Wavelengths"=w264, "Raw Data"=w267) -> (w266:T9)  [unwired: 1 in]
        n145 = Bundle("Array of Wavelengths"=w264, "Raw Data"=w263) -> (w262:T9)  [unwired: 1 in]
        n146 = Build Array(w266, w262) -> (→"UnProcessed Spectra":T1)
        "Spectrum" <- w268
      }
      event #9 {
        n147 = event-data() -> ()  [unwired: 1 in, 5 out]
        n148 = flat-sequence {
          tunnel: w293 -> [w297]
          tunnel: w292 -> [w296]
          tunnel: [w294] -> w290
          tunnel: [w298] -> w289
          tunnel: [w300] -> w291
          tunnel: w289 -> [w301]
          frame #0 {
            n149 = call "SaveData No Objects.vi"("error in (no error)"=w297, "Comments"="Comments", "File Name"="File Name", "Synapse CCD in"=w296) -> ("error out"=w298:errorcluster, "Synapse CCD out"=w294:T5)  [unwired: 6 in]
          }
          frame #1 {
            n150 = call <vilib>:"Simple Error Handler.vi"("error in (no error)"=w301) -> ("error out"=w300:errorcluster)  [unwired: 4 in, 4 out]
            n151 = local write "Export\nPlot"(FALSE) -> ()
          }
        }
      }
      event #10 {
        n152 = event-data() -> ()  [unwired: 1 in, 5 out]
      }
    }
  }
  "error out" <- w1
